vi "AutoRollers.vi"(6 "Override Speed":dbl, 8 "State":dbl, 9 "Close Rollers":i32, 10 "Align":i32, 11 "Mode":i32) -> (1 "Done?":bool)   [LabVIEW 2014]
uses:
  Common Code/Roller Manual Bools.ctl
  Rollers/Really Real Manual Align.ctl
  Rollers/Roller Modes.ctl
  Common Code/Auto Roller Commands.ctl
  Common Code/Roller Mode Enum.ctl
  Robot Global Data.vi
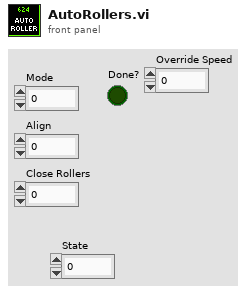
[diagram p1: front panel]
types:
  T1 = typedef "Roller Modes.ctl" = cluster{"Auto Roller Command":T2, "Roller Mode":T3, "Override Intake Speed":dbl}
  T2 = typedef "Auto Roller Commands.ctl" = enum16{"Drag Tote", "Grab Tote", "Idle", "Eject Tote", "Untip Can", "Grab Can"}
  T3 = typedef "Roller Mode Enum.ctl" = enum16{"Manual", "Safe", "Auto"}
  T4 = typedef "Roller Manual Bools.ctl" = cluster{"Manual Claw":bool, "Manual Align":T5, "Left Speed":dbl, "Right Speed":dbl}
  T5 = typedef "Really Real Manual Align.ctl" = enum16{"In", "Left", "Right", "Out", "Idle", "HP Load", "Speeds"}
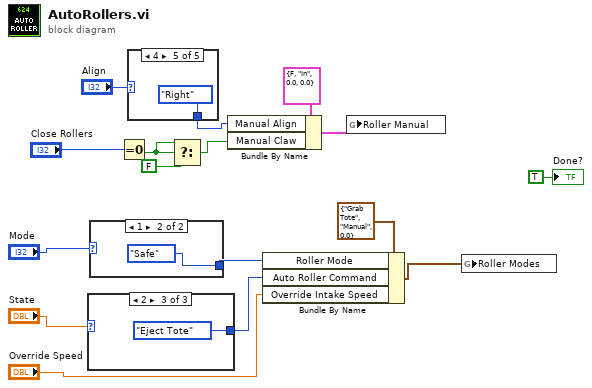
[diagram p0: block diagram]
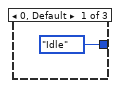
[diagram p2: hidden frame]
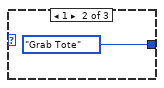
[diagram p3: hidden frame]
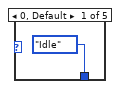
[diagram p4: hidden frame]
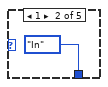
[diagram p5: hidden frame]
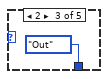
[diagram p6: hidden frame]
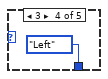
[diagram p7: hidden frame]
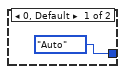
[diagram p8: hidden frame]
diagram:
  n1 = case shown="2" "State" {
    tunnel: [Auto_Roller_Commands."Idle" ("Auto Roller Command") Auto_Roller_Commands."Grab Tote" ("Auto Roller Command") Auto_Roller_Commands."Eject Tote" ("Auto Roller Command")] -> w3
    frame 0, Default {
    }
    frame 1 {
    }
    frame 2 {
    }
  }
  n2 = case shown="1" "Mode" {
    tunnel: [Roller_Mode_Enum."Auto" ("Roller Mode") Roller_Mode_Enum."Safe" ("Roller Mode")] -> w11
    frame 0, Default {
    }
    frame 1 {
    }
  }
  n3 = Equal To 0?(x="Close Rollers") -> (x = 0?=w6:bool)
  n4 = case shown="4" "Align" {
    tunnel: [Really_Real_Manual_Align."Idle" ("Manual Align") Really_Real_Manual_Align."In" ("Manual Align") Really_Real_Manual_Align."Out" ("Manual Align") Really_Real_Manual_Align."Left" ("Manual Align") Really_Real_Manual_Align."Right" ("Manual Align")] -> w9
    frame 0, Default {
    }
    frame 1 {
    }
    frame 2 {
    }
    frame 3 {
    }
    frame 4 {
    }
  }
  n5 = Select(t=w6, s=w6, f=FALSE) -> (s? t:f=w7:bool)
  n6 = Bundle By Name(cluster=T4 {"Manual Claw"=FALSE, "Manual Align"=enum."In", "Left Speed"=0.0, "Right Speed"=0.0} ("Roller Manual"), "Manual Align"=w9, "Manual Claw"=w7) -> (w13:T4)
  n7 = Bundle By Name(cluster=T1 {"Auto Roller Command"=enum."Grab Tote", "Roller Mode"=enum."Manual", "Override Intake Speed"=0.0} ("Roller Modes"), "Roller Mode"=w11, "Auto Roller Command"=w3, "Override Intake Speed"="Override Speed") -> (w14:T1)
  n8 = global write "Robot Global Data.vi" "Roller Manual"(w13) -> ()
  n9 = global write "Robot Global Data.vi" "Roller Modes"(w14) -> ()
  "Done?" <- TRUE ("Done?")
